vi "Set User Password.vi"(0 "User Configuration Manager in":refnum<class "User Configuration Manager.lvclass">, 5 "Username":string, 7 "Current Password":string, 9 "New Password":string, 11 "error in (no error)":errorcluster) -> (4 "User Configuration Manager out":refnum<class "User Configuration Manager.lvclass">, 6 "Found":bool, 15 "error out":errorcluster)   [LabVIEW 2020, in "User Configuration Manager.lvlib" / "User Configuration Manager.lvclass"]
doc: "Sets the password of the user specified by user name."
uses:
  <vilib>/gpm_packages/@cs/user-manager/Source/User Configuration Manager/User Configuration Manager.lvclass
  <vilib>/gpm_packages/@cs/user-manager/Source/User Configuration Manager/User Configuration Manager.lvclass/User Configuration Manager.ctl
  6e98658f-c396-47bf-a1ee-4d1e2e416d22.vi
  4c0e7ab0-d62e-48ee-8387-66e9a9eb6bf5.vi
  <vilib>/gpm_packages/@cs/user-manager/Source/User Configuration Manager/Accessors/Read Linked List Ref .vi
  <vilib>/gpm_packages/@cs/user-manager/Source/User Configuration Manager/Read Encryption Type.vi
  <vilib>/gpm_packages/@cs/linked-list/Source/Linked List/ILinkedList/ILinked List.lvclass
  <vilib>/gpm_packages/@cs/user-manager/Source/iEncryption/iEncryption.lvclass
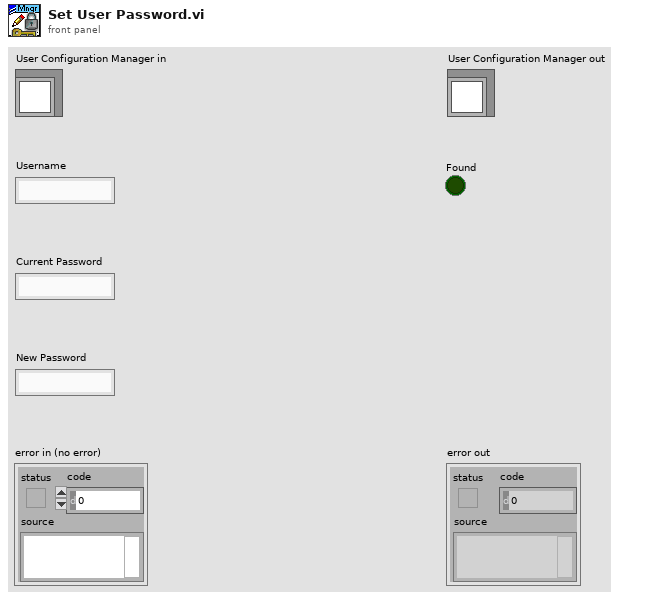
[diagram p1: front panel]
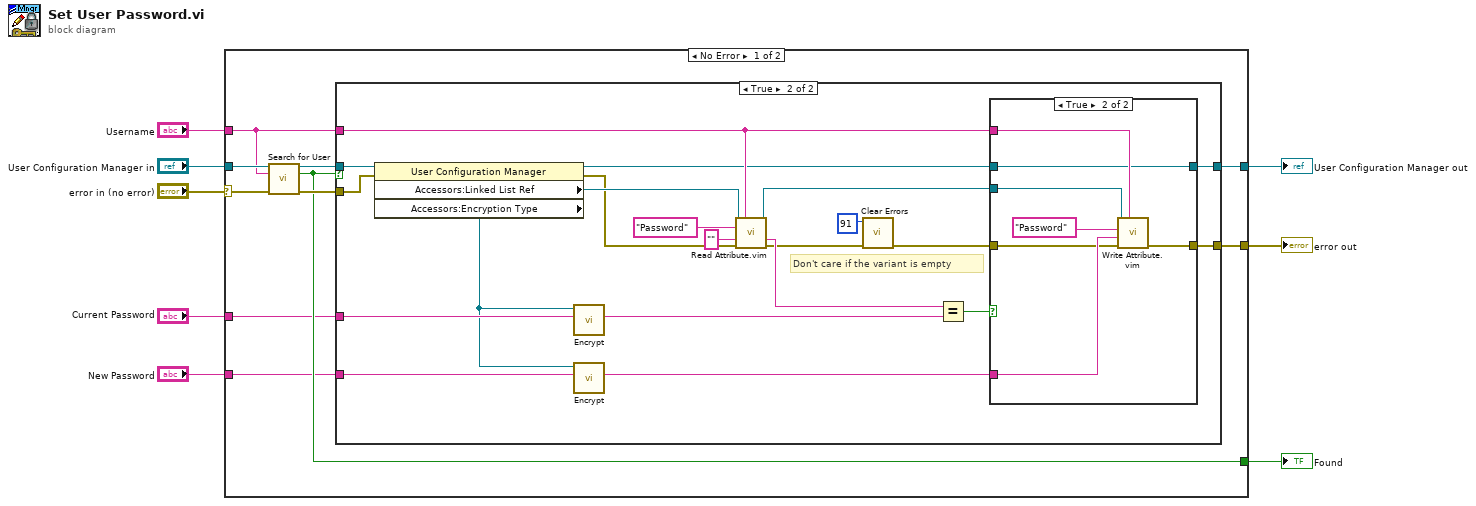
[diagram p0: block diagram]
diagram:
  n1 = case shown="No Error" "error in (no error)" {
    selector: "error in (no error)" -> [w13 w51]
    tunnel: "User Configuration Manager in" -> [w16 w52]
    tunnel: "Username" -> [w9 _]
    tunnel: [w18 w52] -> w5
    tunnel: [w17 w51] -> w4
    tunnel: [w12 _] -> w3
    tunnel: "Current Password" -> [w11 _]
    tunnel: "New Password" -> [w10 _]
    frame No Error {
      n2 = call-dynamic "Search for User.vi"("User Configuration Manager in"=w16, "Username"=w9, "error in (no error)"=w13) -> ("User Configuration Manager out"=w15:refnum<class "User Configuration Manager.lvclass">, "Found"=w12:bool, "error out"=w14:errorcluster)  [unwired: 10 in]
      n3 = case shown="True" w12 {
        tunnel: [w20 w26] -> w18
        tunnel: [w19 w41] -> w17
        tunnel: w15 -> [w20 w40]
        tunnel: w14 -> [w19 w39]
        tunnel: w11 -> [_ w25]
        tunnel: w10 -> [_ w22]
        tunnel: w9 -> [_ w34]
        frame False {
        }
        frame True {
          # "Don't care if the variant is empty"
          n4 = property class="User Configuration Manager"(reference=w40, error in=w39) -> (reference out=w27:refnum<class "User Configuration Manager.lvclass">, error out=w31:errorcluster, "Accessors:Linked List Ref "=w38:refnum<data-value>, "Accessors:Encryption Type"=w23:refnum<class "iEncryption.lvclass">)
          n5 = call-dynamic "Encrypt.vi"("String"=w25, "iEncryption in"=w23) -> ("Encrypted String"=w24:string)  [unwired: 9 in]
          n6 = call-dynamic "Encrypt.vi"("String"=w22, "iEncryption in"=w23) -> ("Encrypted String"=w21:string)  [unwired: 9 in]
          n7 = call "Read Attribute.vim"("Linked List Ref"=w38, "Linked List ID"=w34, "Attribute Name"="Password", "Type"="" ("Attribute Name"), "error in (no error)"=w31) -> ("Linked List Ref out"=w35:refnum<data-value>, "Attribute"=w33:string, "error out"=w30:errorcluster)  [unwired: 5 in, 3 out]
          n8 = call <vilib>:"Clear Errors.vi"("error in (no error)"=w30, "specific error code to clear (0: all)"=91) -> ("error out"=w28:errorcluster)  [unwired: 4 in, 1 out]
          n9 = Equal?(x=w33, y=w24) -> (x = y?=w32:bool)
          n10 = case shown="True" w32 {
            tunnel: [w43 w50] -> w41
            tunnel: w35 -> [_ w49]
            tunnel: w34 -> [_ w48]
            tunnel: w21 -> [_ w47]
            tunnel: w28 -> [w43 w46]
            tunnel: [w42 w45] -> w26
            tunnel: w27 -> [w42 w45]
            frame False {
            }
            frame True {
              n11 = call "Write Attribute.vim"("Linked List ID"=w48, "error in (no error)"=w46, "Attribute"=w47, "Attribute Name"="Password", "Linked List Ref"=w49) -> ("error out"=w50:errorcluster)  [unwired: 3 in, 3 out]
            }
          }
        }
      }
    }
    frame Error {
    }
  }
  "error out" <- w4
  "User Configuration Manager out" <- w5
  "Found" <- w3
